vi "updatePIDConstants.vi"(6 "new k_d":dbl, 8 "error in (no error)":errorcluster, 9 "new k_p":dbl, 10 "new k_i":dbl, 11 "PIDController in":refnum<class "PIDController.lvclass">) -> (0 "error out":errorcluster, 3 "PIDController out":refnum<class "PIDController.lvclass">)   [LabVIEW 2025, in "PIDController.lvclass"]
uses:
  PIDController.lvclass
  PIDController.lvclass/PIDController.ctl
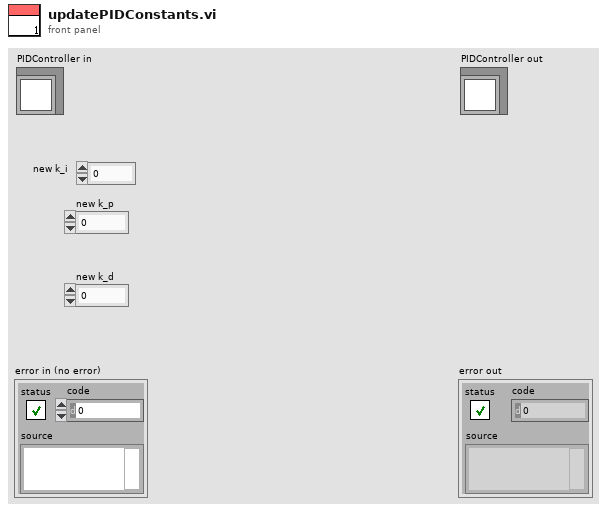
[diagram p1: front panel]
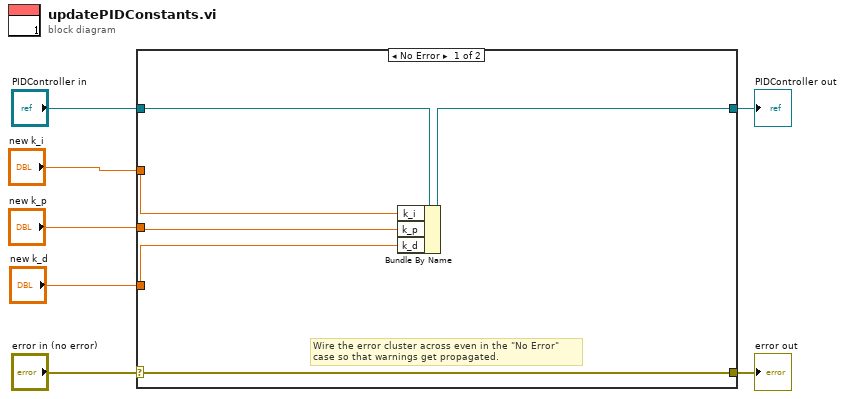
[diagram p0: block diagram]
diagram:
  n1 = case shown="No Error" "error in (no error)" {
    selector: "error in (no error)" -> [w13 w15]
    tunnel: [w13 w15] -> w6
    tunnel: [w12 w14] -> w4
    tunnel: "PIDController in" -> [w9 w14]
    tunnel: "new k_i" -> [w8 _]
    tunnel: "new k_p" -> [w11 _]
    tunnel: "new k_d" -> [w10 _]
    frame No Error {
      # "Wire the error cluster across even in the \"No Error\"\ncase so that warnings get propagated."
      n2 = Bundle By Name(cluster=w9, "k_i"=w8, "k_p"=w11, "k_d"=w10) -> (w12:refnum<class "PIDController.lvclass">)
    }
    frame Error {
    }
  }
  "error out" <- w6
  "PIDController out" <- w4
